vi "Close Sessions VNA.vi"(10 "Instrument Sessions":refnum<k15>[](array[refnum]), 11 "Semiconductor Module Context":T1) -> (0 "error out":errorcluster)   [LabVIEW 2013]
uses:
  <vilib>/NI_TestStand_SemiconductorModule/NI_TestStand_Semiconductor_Module.lvlibp/PinMap/General/SemiconductorModuleContext.ctl
  Pin Map API/VNA Custom Instrument.lvlib
  <vilib>/NI_TestStand_SemiconductorModule/NI_TestStand_Semiconductor_Module.lvlibp
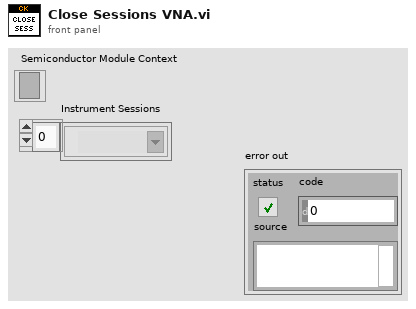
[diagram p1: front panel]
types:
  T1 = typedef "NI_TestStand_Semiconductor_Module.lvlibp/SemiconductorModuleContext.ctl" = refnum<k7>
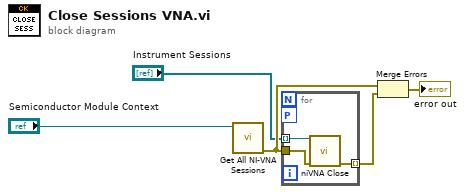
[diagram p0: block diagram]
diagram:
  n1 = call "Get All NI-VNA Sessions.vi"("Semiconductor Module Context"="Semiconductor Module Context") -> ("error out"=w3:errorcluster)  [unwired: 8 in, 2 out]
  n2 = for {
    tunnel: w3 -> [w6]
    tunnel: "Instrument Sessions" -> [w7] mode=indexing
    tunnel: [w8] -> w4 mode=indexing
    workers-P: _ -> [_]
    n3 = call <instrlib>:"niVNA Close.vi"("instrument handle"=w7, "error in"=w6) -> ("error out"=w8:errorcluster)  [unwired: 13 in]
  }
  n4 = Merge Errors(w3, w4) -> (→"error out":errorcluster)
